vi "Exercise 4.5.vi"() -> ()   [LabVIEW 2020]
panel:
  out "Result 2":i32
  out "Result 1":i32
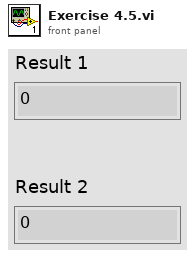
[diagram p1: front panel]
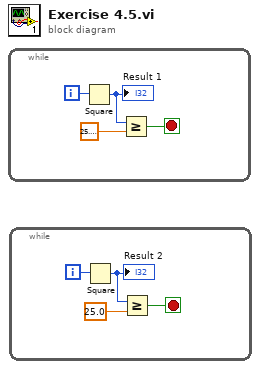
[diagram p0: block diagram]
diagram:
  n1 = while {
    i -> [w4]
    stop <- w3 stop-if-true
    n2 = Square(x=w4) -> (x^2=w2:i32)
    "Result 1" <- w2
    n3 = Greater Or Equal?(x=w2, y=25.00000000001) -> (x >= y?=w3:bool)
  }
  n4 = while {
    i -> [w8]
    stop <- w7 stop-if-true
    n5 = Square(x=w8) -> (x^2=w6:i32)
    "Result 2" <- w6
    n6 = Greater Or Equal?(x=w6, y=25.0) -> (x >= y?=w7:bool)
  }
